vi "PI_TWC-TWS.vi"(7 "TWC?":bool, 8 "Curve_Start_Pixel":u16, 9 "Axis Identifier":string, 10 "Pixel per scan":u16, 11 "Commandset in":string[](array[string])) -> (3 "Commandset out":string[](array[string]))   [LabVIEW 2013]
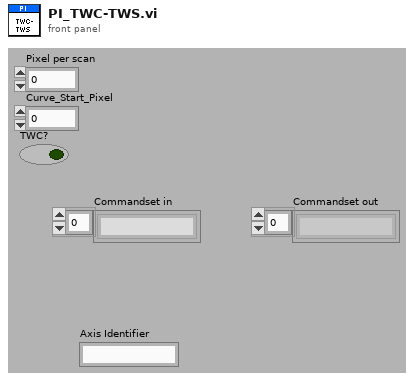
[diagram p1: front panel]
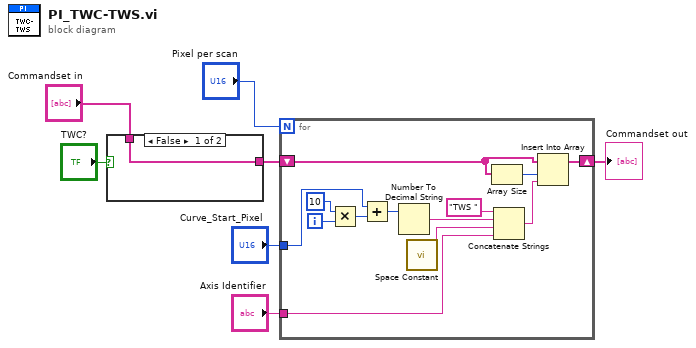
[diagram p0: block diagram]
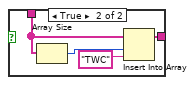
[diagram p2: hidden frame]
diagram:
  n1 = case shown="False" "TWC?" {
    tunnel: "Commandset in" -> [w8 w12]
    tunnel: [w8 w9] -> w3
    frame False {
    }
    frame True {
      n2 = Array Size(array=w12) -> (size(s)=w11:i32)
      n3 = Insert Into Array(array=w12, index=w11, new element="TWC" ("new element/subarray")) -> (w9:string[])
    }
  }
  n4 = for {
    N: "Pixel per scan" -> [_]
    tunnel: "Curve_Start_Pixel" -> [w20]
    shift-right: [w24] -> w6
    shift-left: w3 -> [w18]
    tunnel: "Axis Identifier" -> [w14]
    i -> [w23]
    n5 = Multiply(x=10, y=w23) -> (x*y=w21:i32)
    n6 = Add(x=w20, y=w21) -> (x+y=w15:i32)
    n7 = Number To Decimal String(number=w15) -> (decimal integer string=w13:string)  [unwired: 1 out]
    n8 = call <vilib>:"Space Constant.vi"() -> ("String"=w16:string)
    n9 = Array Size(array=w18) -> (size(s)=w25:i32)
    n10 = Concatenate Strings("TWS " ("new element/subarray"), w13, w16, w14) -> (w17:string)
    n11 = Insert Into Array(array=w18, index=w25, new element=w17) -> (w24:string[])
  }
  "Commandset out" <- w6
